vi "Serial Printer Buffer Handler.vi"(7 "Serials buffer operations":T1(ring), 8 "error in (no error)":errorcluster, 10 "Status":string, 11 "Serial":string) -> (0 "error out":errorcluster, 3 "poped serial":string)   [LabVIEW 2024]
panel:
  out "Buffer":string[][](array[string])
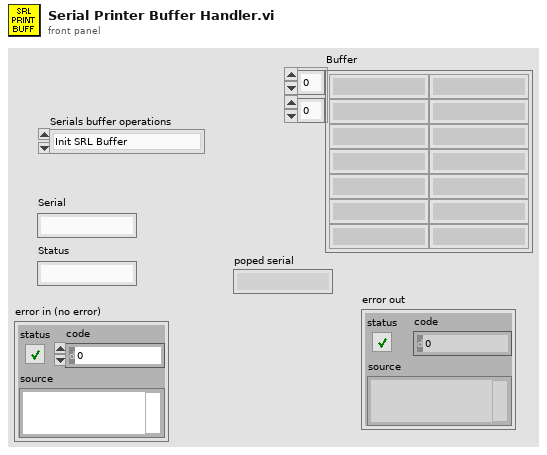
[diagram p1: front panel]
types:
  T1 = enum16{"Init SRL Buffer", "Insert SRL in Buffer", "Insert SRL Status", "Remove SRL from Buffer", "pop serial"}
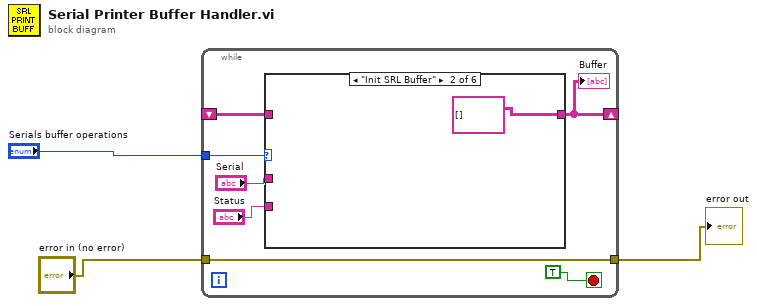
[diagram p0: block diagram]
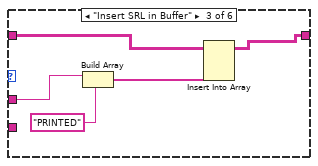
[diagram p3: hidden frame]
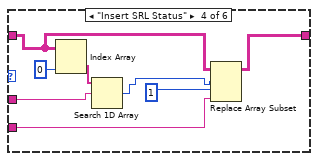
[diagram p4: hidden frame]
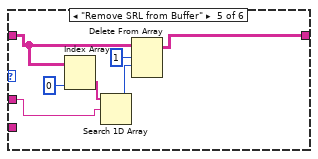
[diagram p5: hidden frame]
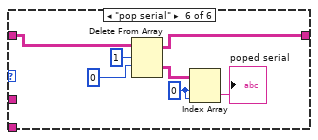
[diagram p6: hidden frame]
diagram:
  n1 = while {
    tunnel: "Serials buffer operations" -> [w9]
    shift-right: [w5] -> _
    shift-left: _ -> [w8]
    tunnel: [w4] -> w2
    tunnel: "error in (no error)" -> [w4]
    stop <- TRUE stop-if-true
    n2 = case shown="\"Init SRL Buffer\"" w9 {
      tunnel: [w11 string[][] [] ("Buffer") w14 w18 w32 w39] -> w5
      tunnel: w8 -> [w11 _ w17 w22 w29 w38]
      tunnel: "Serial" -> [_ _ w13 w23 w28 _]
      tunnel: "Status" -> [_ _ _ w19 _ _]
      frame Default {
      }
      frame "Init SRL Buffer" {
      }
      frame "Insert SRL in Buffer" {
        n3 = Build Array(w13, "PRINTED" ("element")) -> (w15:string[])
        n4 = Insert Into Array(array=w17, new element=w15) -> (w14:string[][])  [unwired: 2 in]
      }
      frame "Insert SRL Status" {
        n5 = Index Array(array=w22, index (col)=0 ("disabled index (col)")) -> (element=w24:string[])  [unwired: 1 in]
        n6 = Search 1D Array(1D array=w24, element=w23) -> (index of element=w21:i32)  [unwired: 1 in]
        n7 = Replace Array Subset(array=w22, new element=w19, index (row)=w21, index (col)=1) -> (w18:string[][])
      }
      frame "Remove SRL from Buffer" {
        n8 = Index Array(array=w29, index (col)=0 ("disabled index (col)")) -> (element=w30:string[])  [unwired: 1 in]
        n9 = Search 1D Array(1D array=w30, element=w28) -> (index of element=w27:i32)  [unwired: 1 in]
        n10 = Delete From Array(array=w29, length=1, index (row)=w27) -> (array with subset deleted=w32:string[][])  [unwired: 1 in, 1 out]
      }
      frame "pop serial" {
        w34 = 0 ("index (row)")
        n11 = Delete From Array(array=w38, length=1, index (row)=0) -> (deleted portion=w35:string[][], array with subset deleted=w39:string[][])  [unwired: 1 in]
        n12 = Index Array(array=w35, index (row)=w34, index (col)=w34) -> (element=→"poped serial":string)
      }
    }
    "Buffer" <- w5
  }
  "error out" <- w2
